vi "数据接收处理.vi"(0 "字符串":string) -> (1 "ADC":u16, 2 "ENC":u16)   [LabVIEW 2022 SP3]
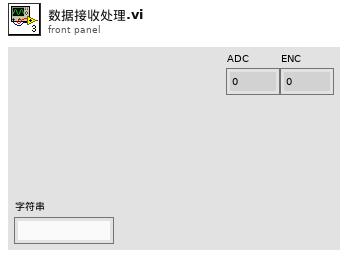
[diagram p1: front panel]
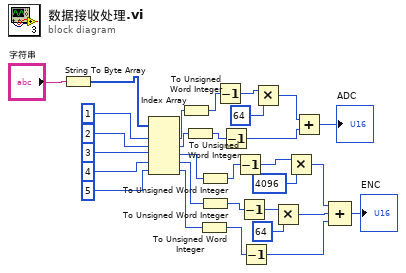
[diagram p0: block diagram]
diagram:
  n1 = String To Byte Array(string="字符串") -> (unsigned byte array=w5:u8[])
  n2 = Index Array(array=w5, index #1=1 ("索引"), index #2=2 ("索引"), index #3=3 ("索引"), index #4=4 ("索引"), index #5=5 ("索引")) -> (element #1=w15:u8, element #2=w17:u8, element #3=w20:u8, element #4=w21:u8, element #5=w22:u8)
  n3 = To Unsigned Word Integer(number=w15) -> (unsigned 16bit integer=w16:u16)
  n4 = To Unsigned Word Integer(number=w17) -> (unsigned 16bit integer=w18:u16)
  n5 = To Unsigned Word Integer(number=w22) -> (unsigned 16bit integer=w25:u16)
  n6 = To Unsigned Word Integer(number=w20) -> (unsigned 16bit integer=w23:u16)
  n7 = To Unsigned Word Integer(number=w21) -> (unsigned 16bit integer=w24:u16)
  n8 = Decrement(x=w16) -> (x-1=w4:u16)
  n9 = Decrement(x=w18) -> (x-1=w19:u16)
  n10 = Decrement(x=w23) -> (x-1=w26:u16)
  n11 = Decrement(x=w24) -> (x-1=w27:u16)
  n12 = Decrement(x=w25) -> (x-1=w30:u16)
  n13 = Multiply(x=w4, y=u16 64) -> (x*y=w3:u16)
  n14 = Multiply(x=w27, y=u16 64) -> (x*y=w29:u16)
  n15 = Multiply(x=w26, y=u16 4096) -> (x*y=w28:u16)
  n16 = Add(x=w3, y=w19) -> (x+y=→"ADC":u16)
  n17 = Compound Arithmetic op=ADD(w28, w29, w30) -> (→"ENC":u16)
